vi "visa_read.vi"() -> ()   [LabVIEW 2011]
panel:
  in  "Input":string="KRDG? a\\n"
  out "Output":string
  out "error out":errorcluster
  in  "VISA resource name":refnum<visa-resource-name>
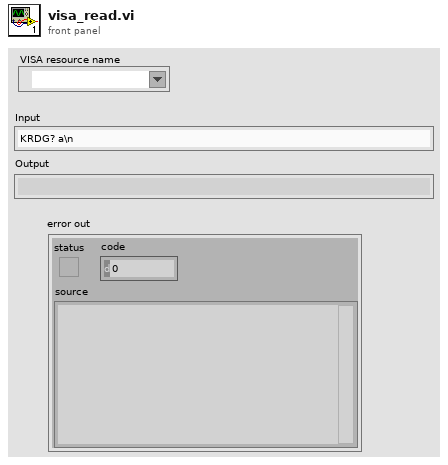
[diagram p1: front panel]
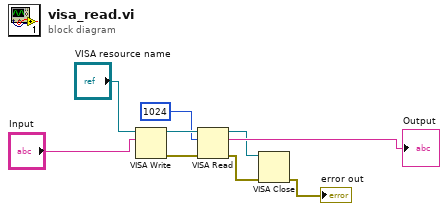
[diagram p0: block diagram]
diagram:
  n1 = VISA Write(VISA resource name="VISA resource name", write buffer="Input") -> (VISA resource name out=w8:refnum<visa-resource-name>, error out=w9:errorcluster)  [unwired: 1 in, 1 out]
  n2 = VISA Read(VISA resource name=w8, byte count=1024, error in (no error)=w9) -> (VISA resource name out=w1:refnum<visa-resource-name>, read buffer=→"Output":string, error out=w3:errorcluster)  [unwired: 1 out]
  n3 = VISA Close(VISA resource name=w1, error in (no error)=w3) -> (error out=→"error out":errorcluster)
